vi "read control value.vi"(6 "call chain index (1)":i32=1, 7 "vi ref (caller)":refnum<vi>, 8 "error in (no error)":errorcluster, 11 "label":string) -> (0 "error out":errorcluster, 3 "value":variant)   [LabVIEW 2024, in "controls manager.lvlib"]
uses:
  controls manager.lvlib
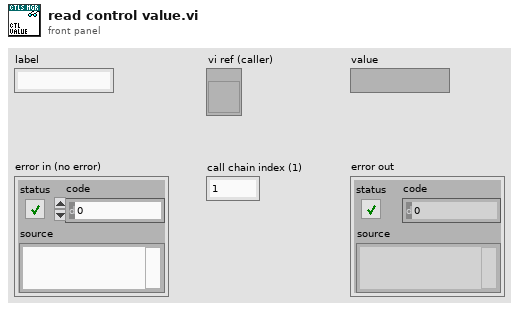
[diagram p1: front panel]
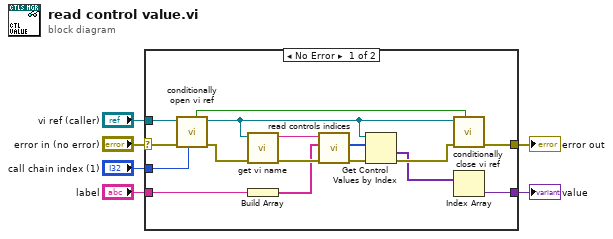
[diagram p0: block diagram]
diagram:
  n1 = case shown="No Error" "error in (no error)" {
    selector: "error in (no error)" -> [w21 w23]
    tunnel: [w18 w23] -> w6
    tunnel: "vi ref (caller)" -> [w15 _]
    tunnel: "call chain index (1)" -> [w14 _]
    tunnel: "label" -> [w13 _]
    tunnel: [w7 _] -> w1
    frame No Error {
      n2 = call "conditionally open vi ref.vi"("call chain index (1)"=w14, "error in (no error)"=w21, "vi ref in"=w15) -> ("error out"=w20:errorcluster, "vi ref out"=w10:refnum<vi>, "new ref?"=w17:bool)  [unwired: 6 in]
      n3 = call "get vi name.vi"("error in (no error)"=w20, "vi ref"=w10) -> ("error out"=w22:errorcluster, "vi name"=w16:string)  [unwired: 8 in]
      n4 = Build Array(w13) -> (w9:string[])
      n5 = call "read controls indices.vi"("error in (no error)"=w22, "labels"=w9, "id"=w16) -> ("error out"=w19:errorcluster, "indices"=w11:i32[])  [unwired: 7 in]
      n6 = Get Control Values by Index(0:w10, 1:w11, 3:w19) -> (10:w8:variant[], 11:w12:errorcluster)
      n7 = call "conditionally close vi ref.vi"("new ref?"=w17, "error in (no error)"=w12, "vi ref"=w10) -> ("error out"=w18:errorcluster)  [unwired: 8 in]
      n8 = Index Array(array=w8) -> (element=w7:variant)  [unwired: 1 in]
    }
    frame Error {
    }
  }
  "error out" <- w6
  "value" <- w1
